vi "xijk_calc_eijk_xijk.vi"(5 "spectra parameters in":T2={"Booleans"={"Unknown detector"=FALSE, "Dual band filters"=FALSE, "Dual emission by cubes"=FALSE, "FRET"=FALSE}, "Integers"={"Light source"=0, "Number of fluorophores"=0, "Wavelength of laser (nm) 1"=0, "Broadness of laser (nm) 1"=0.0, "Wavelength of laser (nm) 2"=0, "Broadness of laser (nm) 2"=0.0, "Template"=1}, "Doubles"={"Molar extinction 1"=1.0, "Molar extinction 2"=1.0, "Quantum efficiency 1"=1.0, "Quantum efficiency 2"=1.0}}, 7 "spectra in":T3, 8 "Effective spectral emission 2":sgl[](array[numeric]), 9 "Effective spectral excitation 2":sgl[](array[numeric]), 10 "Effective spectral emission 1":sgl[](array[numeric]), 11 "Effective spectral excitation 1":sgl[](array[numeric])) -> (3 "output cluster":T1)   [LabVIEW 2009]
uses:
  Type Def/spectrum_table_control.ctl
  Type Def/spectra_parameters.ctl
  Type Def/xijk_cluster.ctl
  <vilib>/Analysis/8numeric.llb/1D Numeric Integration.vi
  <vilib>/Analysis/NI_AALPro.lvlib
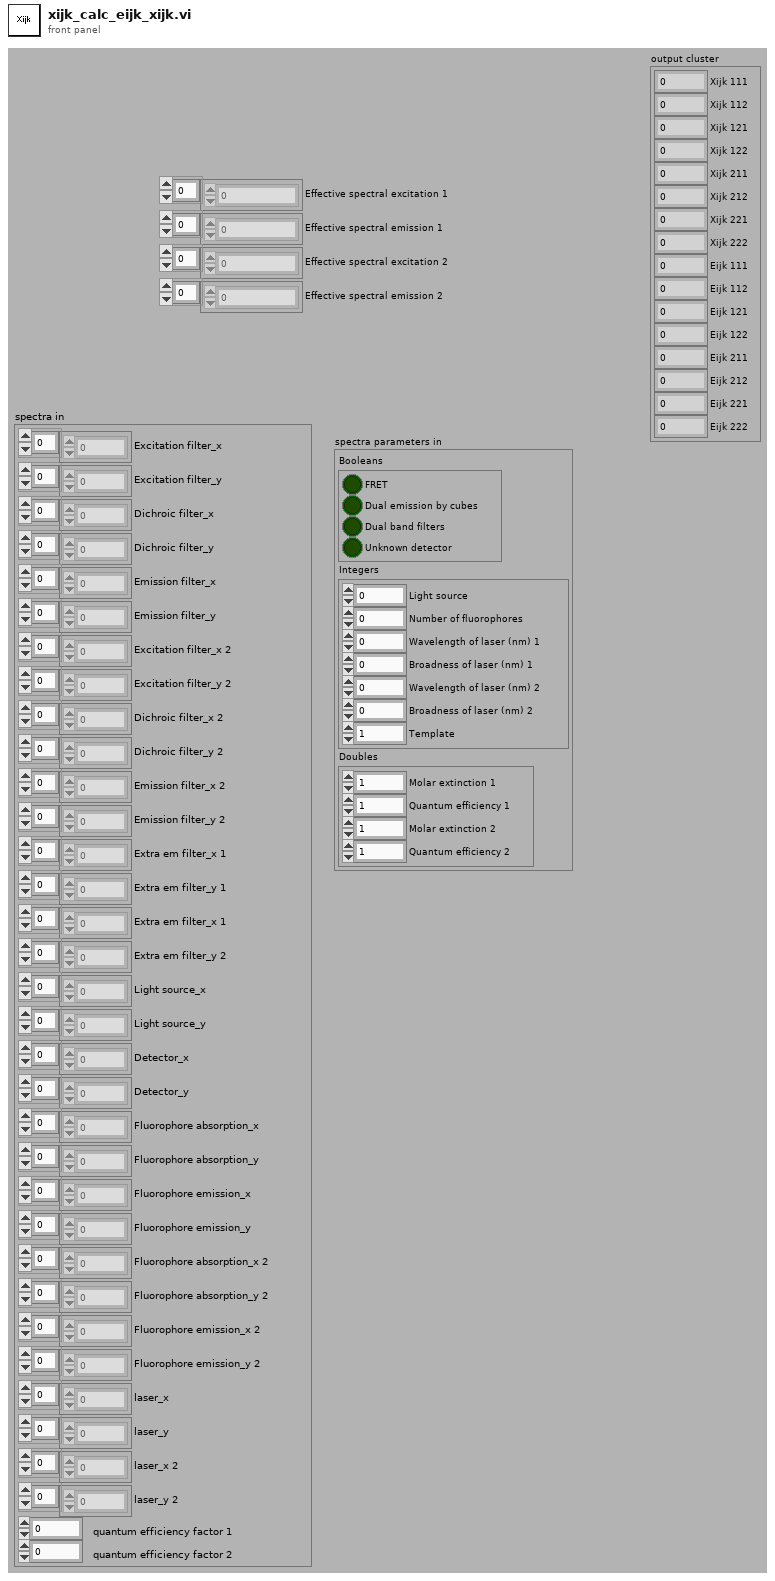
[diagram p1: front panel]
types:
  T1 = typedef "xijk_cluster.ctl" = cluster{"Xijk 111":sgl, "Xijk 112":sgl, "Xijk 121":sgl, "Xijk 122":sgl, "Xijk 211":sgl, "Xijk 212":sgl, "Xijk 221":sgl, "Xijk 222":sgl, "Eijk 111":sgl, "Eijk 112":sgl, "Eijk 121":sgl, "Eijk 122":sgl, "Eijk 211":sgl, "Eijk 212":sgl, "Eijk 221":sgl, "Eijk 222":sgl}
  T2 = typedef "spectra_parameters.ctl" = cluster{"Booleans":cluster{"Unknown detector":bool, "Dual band filters":bool, "Dual emission by cubes":bool, "FRET":bool}, "Integers":cluster{"Light source":u16, "Number of fluorophores":u16, "Wavelength of laser (nm) 1":u16, "Broadness of laser (nm) 1":sgl, "Wavelength of laser (nm) 2":u16, "Broadness of laser (nm) 2":sgl, "Template":u16}, "Doubles":cluster{"Molar extinction 1":sgl, "Molar extinction 2":sgl, "Quantum efficiency 1":sgl, "Quantum efficiency 2":sgl}}
  T3 = typedef "spectrum_table_control.ctl" = cluster{"Excitation filter_x":i16[], "Excitation filter_y":sgl[], "Dichroic filter_x":i16[], "Dichroic filter_y":sgl[], "Emission filter_x":i16[], "Emission filter_y":sgl[], "Excitation filter_x 2":i16[], "Excitation filter_y 2":sgl[], "Dichroic filter_x 2":i16[], "Dichroic filter_y 2":sgl[], "Emission filter_x 2":i16[], "Emission filter_y 2":sgl[], "Extra em filter_x 1":i16[], "Extra em filter_y 1":sgl[], "Extra em filter_x 1":i16[], "Extra em filter_y 2":sgl[], "Light source_x":i16[], "Light source_y":sgl[], "Detector_x":i16[], "Detector_y":sgl[], "Fluorophore absorption_x":i16[], "Fluorophore absorption_y":sgl[], "Fluorophore emission_x":i16[], "Fluorophore emission_y":sgl[], "Fluorophore absorption_x 2":i16[], "Fluorophore absorption_y 2":sgl[], "Fluorophore emission_x 2":i16[], "Fluorophore emission_y 2":sgl[], "laser_x":i16[], "laser_y":sgl[], "laser_x 2":i16[], "laser_y 2":sgl[], "quantum efficiency factor 1":sgl, "quantum efficiency factor 2":sgl}
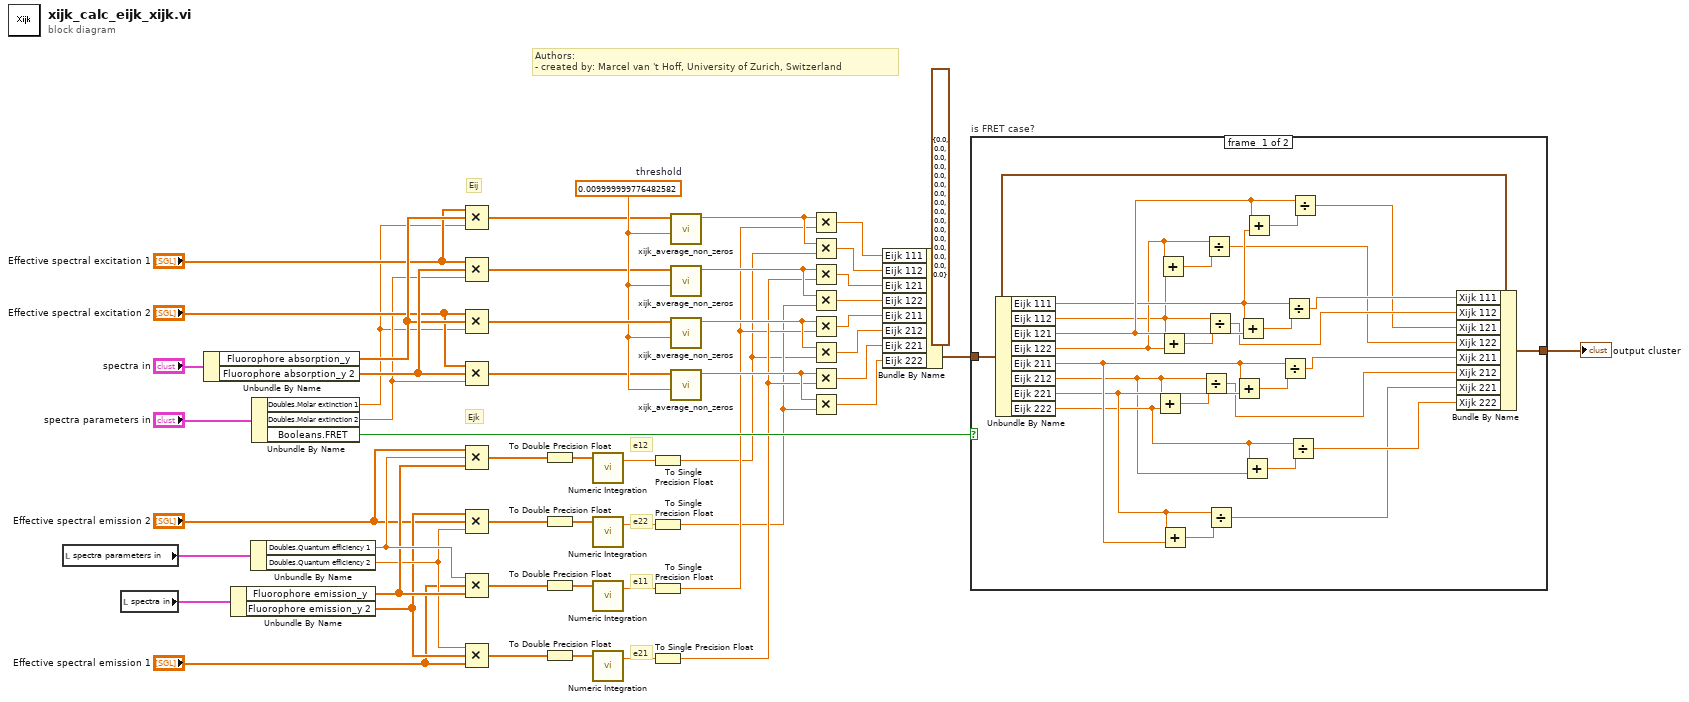
[diagram p0: block diagram]
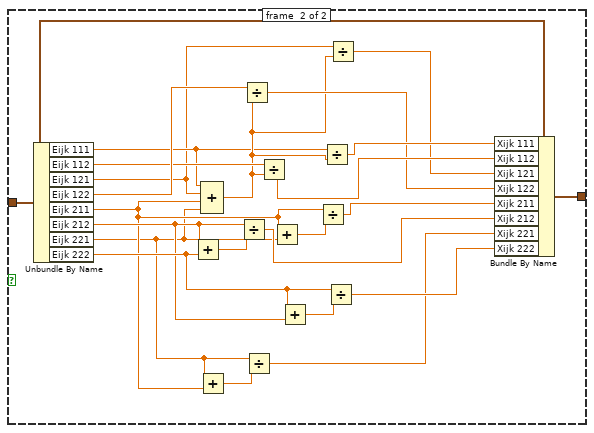
[diagram p2: hidden frame]
diagram:
  w34 = sgl 0.01  # threshold
  # "Ejk"
  # "Eij"
  # "Authors: \n- created by: Marcel van 't Hoff, University of Zurich, Switzerland"
  # "e21"
  # "e11"
  # "e22"
  # "e12"
  n1 = local read "spectra parameters in"() -> (w49:T2)
  n2 = local read "spectra in"() -> (w50:T3)
  n3 = Unbundle By Name("spectra in") -> ("Fluorophore absorption_y"=w44:sgl[], "Fluorophore absorption_y 2"=w51:sgl[])
  n4 = Unbundle By Name(w50) -> ("Fluorophore emission_y"=w47:sgl[], "Fluorophore emission_y 2"=w45:sgl[])
  n5 = Unbundle By Name(w49) -> ("Doubles.Quantum efficiency 1"=w48:sgl, "Doubles.Quantum efficiency 2"=w46:sgl)
  n6 = Unbundle By Name("spectra parameters in") -> ("Doubles.Molar extinction 1"=w36:sgl, "Doubles.Molar extinction 2"=w37:sgl, "Booleans.FRET"=w42:bool)
  n7 = Compound Arithmetic op=MULTIPLY("Effective spectral excitation 1", w44, w36) -> (w19:sgl[])
  n8 = Compound Arithmetic op=MULTIPLY("Effective spectral excitation 1", w51, w37) -> (w18:sgl[])
  n9 = Compound Arithmetic op=MULTIPLY("Effective spectral excitation 2", w44, w36) -> (w35:sgl[])
  n10 = Compound Arithmetic op=MULTIPLY("Effective spectral excitation 2", w51, w37) -> (w20:sgl[])
  n11 = Compound Arithmetic op=MULTIPLY("Effective spectral emission 2", w48, w47) -> (w17:sgl[])
  n12 = Compound Arithmetic op=MULTIPLY(w45, "Effective spectral emission 2", w46) -> (w15:sgl[])
  n13 = Compound Arithmetic op=MULTIPLY(w48, "Effective spectral emission 1", w47) -> (w13:sgl[])
  n14 = Compound Arithmetic op=MULTIPLY(w46, w45, "Effective spectral emission 1") -> (w11:sgl[])
  n15 = To Double Precision Float(number=w17) -> (double precision float=w16:dbl[])
  n16 = To Double Precision Float(number=w15) -> (double precision float=w14:dbl[])
  n17 = To Double Precision Float(number=w13) -> (double precision float=w12:dbl[])
  n18 = To Double Precision Float(number=w11) -> (double precision float=w10:dbl[])
  n19 = call-poly <vilib>:"Numeric Integration.vi"("Input Array"=w16) -> ("result"=w3:dbl)  [unwired: 2 in, 1 out]
  n20 = call-poly <vilib>:"Numeric Integration.vi"("Input Array"=w14) -> ("result"=w5:dbl)  [unwired: 2 in, 1 out]
  n21 = call-poly <vilib>:"Numeric Integration.vi"("Input Array"=w12) -> ("result"=w7:dbl)  [unwired: 2 in, 1 out]
  n22 = call-poly <vilib>:"Numeric Integration.vi"("Input Array"=w10) -> ("result"=w9:dbl)  [unwired: 2 in, 1 out]
  n23 = To Single Precision Float(number=w3) -> (single precision float=w2:sgl)
  n24 = To Single Precision Float(number=w5) -> (single precision float=w4:sgl)
  n25 = To Single Precision Float(number=w7) -> (single precision float=w6:sgl)
  n26 = To Single Precision Float(number=w9) -> (single precision float=w8:sgl)
  n27 = call "xijk_average_non_zeros.vi"("threshold"=w34, "array in"=w19) -> ("average over non-zeros"=w30:sgl)  [unwired: 9 in]
  n28 = call "xijk_average_non_zeros.vi"("threshold"=w34, "array in"=w18) -> ("average over non-zeros"=w27:sgl)  [unwired: 9 in]
  n29 = call "xijk_average_non_zeros.vi"("threshold"=w34, "array in"=w35) -> ("average over non-zeros"=w24:sgl)  [unwired: 9 in]
  n30 = call "xijk_average_non_zeros.vi"("threshold"=w34, "array in"=w20) -> ("average over non-zeros"=w21:sgl)  [unwired: 9 in]
  n31 = Multiply(x=w30, y=w6) -> (x*y=w32:sgl)
  n32 = Multiply(x=w30, y=w2) -> (x*y=w31:sgl)
  n33 = Multiply(x=w27, y=w8) -> (x*y=w29:sgl)
  n34 = Multiply(x=w27, y=w4) -> (x*y=w28:sgl)
  n35 = Multiply(x=w24, y=w6) -> (x*y=w26:sgl)
  n36 = Multiply(x=w24, y=w2) -> (x*y=w25:sgl)
  n37 = Multiply(x=w21, y=w8) -> (x*y=w23:sgl)
  n38 = Multiply(x=w21, y=w4) -> (x*y=w22:sgl)
  n39 = Bundle By Name(cluster=T1 {"Xijk 111"=0.0, "Xijk 112"=0.0, "Xijk 121"=0.0, "Xijk 122"=0.0, "Xijk 211"=0.0, "Xijk 212"=0.0, "Xijk 221"=0.0, "Xijk 222"=0.0, "Eijk 111"=0.0, "Eijk 112"=0.0, "Eijk 121"=0.0, "Eijk 122"=0.0, "Eijk 211"=0.0, "Eijk 212"=0.0, "Eijk 221"=0.0, "Eijk 222"=0.0} ("Xijk output cluster"), "Eijk 111"=w32, "Eijk 112"=w31, "Eijk 121"=w29, "Eijk 122"=w28, "Eijk 211"=w26, "Eijk 212"=w25, "Eijk 221"=w23, "Eijk 222"=w22) -> (w1:T1)
  n40 = case "is FRET case?" shown="True" w42 {
    tunnel: w1 -> [w55 w88]
    tunnel: [w54 w87] -> w43
    frame #0 {
      n41 = Unbundle By Name(w55) -> ("Eijk 111"=w73:sgl, "Eijk 112"=w70:sgl, "Eijk 121"=w74:sgl, "Eijk 122"=w71:sgl, "Eijk 211"=w67:sgl, "Eijk 212"=w64:sgl, "Eijk 221"=w66:sgl, "Eijk 222"=w65:sgl)
      n42 = Add(x=w64, y=w65) -> (x+y=w76:sgl)
      n43 = Add(x=w71, y=w70) -> (x+y=w72:sgl)
      n44 = Add(x=w70, y=w71) -> (x+y=w77:sgl)
      n45 = Add(x=w66, y=w67) -> (x+y=w69:sgl)
      n46 = Divide(x=w64, y=w76) -> (x/y=w60:sgl)
      n47 = Divide(x=w71, y=w72) -> (x/y=w58:sgl)
      n48 = Divide(x=w70, y=w77) -> (x/y=w62:sgl)
      n49 = Divide(x=w66, y=w69) -> (x/y=w56:sgl)
      n50 = Add(x=w67, y=w66) -> (x+y=w75:sgl)
      n51 = Add(x=w73, y=w74) -> (x+y=w79:sgl)
      n52 = Add(x=w65, y=w64) -> (x+y=w68:sgl)
      n53 = Add(x=w74, y=w73) -> (x+y=w78:sgl)
      n54 = Divide(x=w67, y=w75) -> (x/y=w61:sgl)
      n55 = Divide(x=w73, y=w79) -> (x/y=w63:sgl)
      n56 = Divide(x=w65, y=w68) -> (x/y=w57:sgl)
      n57 = Divide(x=w74, y=w78) -> (x/y=w59:sgl)
      n58 = Bundle By Name(cluster=w55, "Xijk 111"=w63, "Xijk 112"=w62, "Xijk 121"=w59, "Xijk 122"=w58, "Xijk 211"=w61, "Xijk 212"=w60, "Xijk 221"=w56, "Xijk 222"=w57) -> (w54:T1)
    }
    frame #1 {
      n59 = Unbundle By Name(w88) -> ("Eijk 111"=w83:sgl, "Eijk 112"=w99:sgl, "Eijk 121"=w82:sgl, "Eijk 122"=w100:sgl, "Eijk 211"=w81:sgl, "Eijk 212"=w85:sgl, "Eijk 221"=w80:sgl, "Eijk 222"=w86:sgl)
      n60 = Add(x=w85, y=w86) -> (x+y=w102:sgl)
      n61 = Add(x=w80, y=w81) -> (x+y=w98:sgl)
      n62 = Compound Arithmetic op=ADD(w83, w82, w81, w80) -> (w84:sgl)
      n63 = Divide(x=w85, y=w102) -> (x/y=w93:sgl)
      n64 = Divide(x=w100, y=w84) -> (x/y=w91:sgl)
      n65 = Divide(x=w80, y=w98) -> (x/y=w89:sgl)
      n66 = Divide(x=w99, y=w84) -> (x/y=w95:sgl)
      n67 = Add(x=w81, y=w80) -> (x+y=w101:sgl)
      n68 = Add(x=w86, y=w85) -> (x+y=w97:sgl)
      n69 = Divide(x=w81, y=w101) -> (x/y=w94:sgl)
      n70 = Divide(x=w83, y=w84) -> (x/y=w96:sgl)
      n71 = Divide(x=w86, y=w97) -> (x/y=w90:sgl)
      n72 = Divide(x=w82, y=w84) -> (x/y=w92:sgl)
      n73 = Bundle By Name(cluster=w88, "Xijk 111"=w96, "Xijk 112"=w95, "Xijk 121"=w92, "Xijk 122"=w91, "Xijk 211"=w94, "Xijk 212"=w93, "Xijk 221"=w89, "Xijk 222"=w90) -> (w87:T1)
    }
  }
  "output cluster" <- w43
